vi "InitializeArrays1.vi"(0 "Numbers of frames":i32) -> (1 "X,Y":dbl[][](array[numeric]), 2 "X,Y,dX,dY (NN)":dbl[][](array[numeric]), 3 "Area particles (X,Y)":dbl[][](array[numeric]), 4 "X,Y,dX,dY (Processed)":dbl[][](array[numeric]))   [LabVIEW 2013]
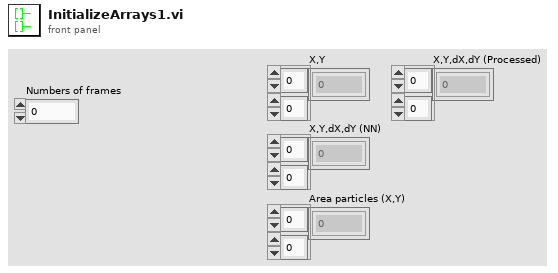
[diagram p1: front panel]
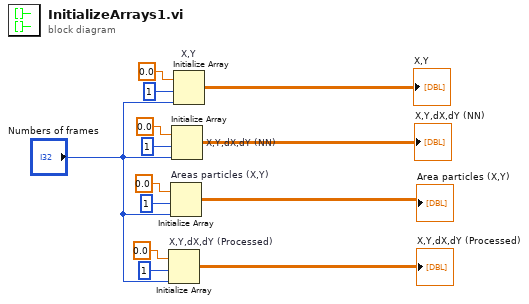
[diagram p0: block diagram]
diagram:
  n1 = Initialize Array "X,Y,dX,dY (Processed)"(0.0 ("element"), 1 ("dimension size"), "Numbers of frames") -> (→"X,Y,dX,dY (Processed)":dbl[][])
  n2 = Initialize Array "Areas particles (X,Y)"(0.0 ("element"), 1 ("dimension size"), "Numbers of frames") -> (→"Area particles (X,Y)":dbl[][])
  n3 = Initialize Array "X,Y,dX,dY (NN)"(0.0 ("element"), 1 ("dimension size"), "Numbers of frames") -> (→"X,Y,dX,dY (NN)":dbl[][])
  n4 = Initialize Array "X,Y"(0.0 ("element"), 1 ("dimension size"), "Numbers of frames") -> (→"X,Y":dbl[][])
